vi "Find Test and Suite Index.vi"(8 "error in (no error)":errorcluster, 11 "Linker.Read Info From File":T2(array[cluster])) -> (0 "error out":errorcluster, 2 "Define Test index":i32, 3 "Define Test Suite index":i32)   [LabVIEW 2013, in "Unit Tests for Runner.lvclass"]
uses:
  Unit Tests for Runner.lvclass
  <vilib>/Utility/lvfile.llb/LVFileType.ctl
  classes/Test/Define Test.vi
  classes/Test Suite/Define Test Suite.vi
  classes/Test/Test.lvclass
  classes/Test Suite/Test Suite.lvclass
  <vilib>/Utility/lvfile.llb/NI_FileType.lvlib
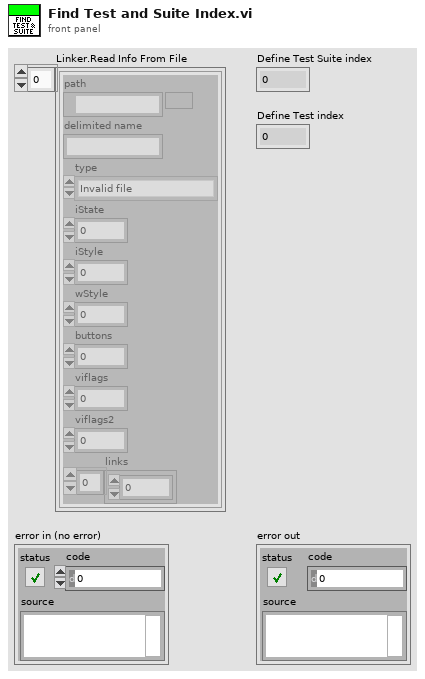
[diagram p1: front panel]
types:
  T1 = typedef "NI_FileType.lvlib/LVFileType.ctl" = enum32{"Invalid file", "Unknown type", "Instrument", "Control", "Polymorphic VI", "Project", "Library", "LVClass", "XControl", "XNode", "Shared library", ".NET assembly", "ActiveX interface", "CIN", "Run-time menu", "Palette menu", "Help file", "LLB", "XNode Edit Dependency", "Class Private Data Control", "Statechart", "MathScript .m file", "Ladder Diagram", "LVLibp", "XNode Build Dependency"}
  T2 = cluster{"path":path, "delimited name":string, "type":T1, "iState":u32, "iStyle":u16, "wStyle":u16, "buttons":u16, "viflags":u32, "viflags2":u32, "links":u32[]}[]
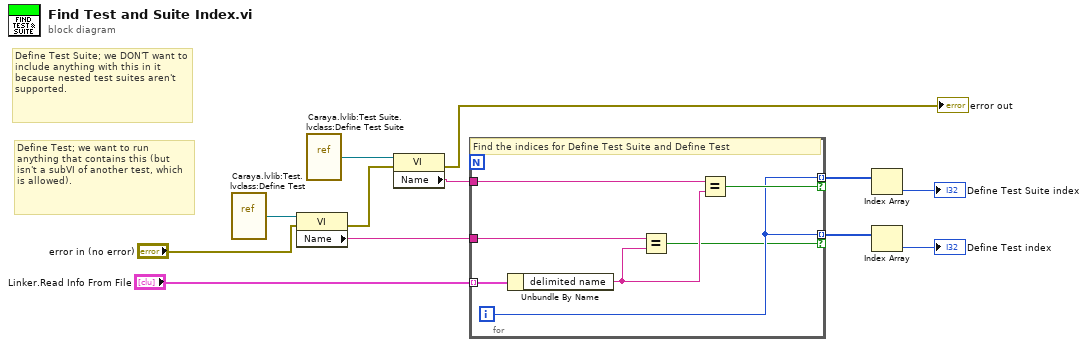
[diagram p0: block diagram]
diagram:
  # "Define Test; we want to run anything that contains this (but isn't a subVI of another test, which is allowed)."
  # "Define Test Suite; we DON'T want to include anything with this in it because nested test suites aren't supported."
  n1 = vi-ref "Caraya.lvlib:Test.lvclass:Define Test.vi"() -> (w1:refnum<vi>)
  n2 = property class="VI"(reference=w1, error in="error in (no error)") -> (error out=w4:errorcluster, "Name"=w6:string)  [unwired: 1 out]
  n3 = vi-ref "Caraya.lvlib:Test Suite.lvclass:Define Test Suite.vi"() -> (w3:refnum<vi>)
  n4 = property class="VI"(reference=w3, error in=w4) -> (error out=→"error out":errorcluster, "Name"=w5:string)  [unwired: 1 out]
  n5 = for {
    tunnel: "Linker.Read Info From File" -> [w19] mode=indexing
    tunnel: w5 -> [w17]
    tunnel: w6 -> [w18]
    tunnel: [w14] -> w7 mode=indexing if=w15
    tunnel: [w14] -> w8 mode=indexing if=w13
    i -> [w14]
    # "Find the indices for Define Test Suite and Define Test"
    n6 = Unbundle By Name(w19) -> ("delimited name"=w16:string)
    n7 = Equal?(x=w18, y=w16) -> (x = y?=w13:bool)
    n8 = Equal?(x=w17, y=w16) -> (x = y?=w15:bool)
  }
  n9 = Index Array(array=w7) -> (element=→"Define Test Suite index":i32)  [unwired: 1 in]
  n10 = Index Array(array=w8) -> (element=→"Define Test index":i32)  [unwired: 1 in]
